vi "XY to Rtheta.vi"(2 "Y":dbl, 3 "X":dbl) -> (0 "theta (deg)":dbl, 1 "R":dbl)   [LabVIEW 2009]
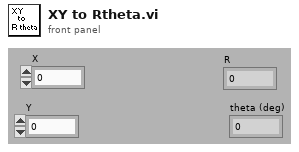
[diagram p1: front panel]
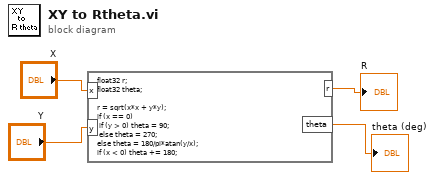
[diagram p0: block diagram]
diagram:
  n1 = formula code="float32 r;\nfloat32 theta;\n\nr = sqrt(x*x + y*y);\nif (x == 0) \n if (y > 0) theta = 90;\n else theta = 270;\nelse theta = 180/pi*atan(y/x);\nif (x < 0) theta += 180;"("x"="X", "y"="Y") -> ("r"=→"R":sgl, "theta"=→"theta (deg)":sgl)
